vi "build memory.vi"(8 "error in (no error)":errorcluster caption="에러 입력(에러 없음)", 10 "WF List":T1[](array[typedef]), 11 "Haptic IC 입력":refnum<class "Haptic IC.lvclass">) -> (0 "error out":errorcluster caption="에러 출력", 1 "memory data by wf":cluster{"Header":u8[], "Data":u8[]}[](array[cluster]), 2 "full memory data":u8[](array[numeric]), 3 "Haptic IC 출력":refnum<class "Haptic IC.lvclass">)   [LabVIEW 2020, in "Haptic IC.lvclass"]
uses:
  Haptic IC.lvclass
  SubVIs/Waveform Editor/Controls/(Ctrl)Waveform Editor_WF List.ctl
  Waveform Obj Class/Waveform Obj/Waveform Obj.lvclass
  Waveform Obj Class/Waveform Obj/Waveform Obj.lvclass/Waveform Obj.ctl
  Waveform Obj Class/Waveform Obj/Accessors/Read sampling rate.vi
  Waveform Obj Class/Waveform Obj/Accessors/Read voltage range.vi
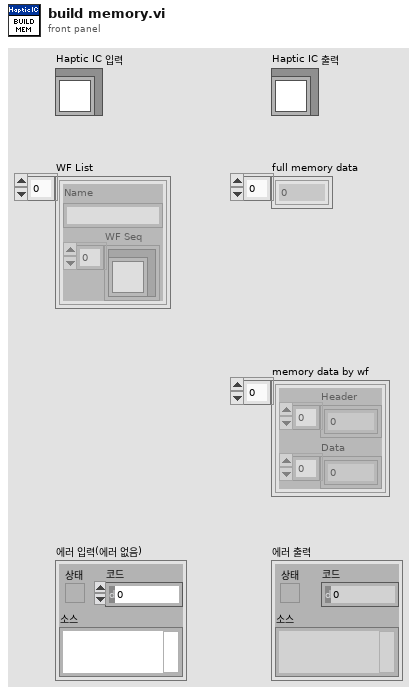
[diagram p1: front panel]
types:
  T1 = typedef "(Ctrl)Waveform Editor_WF List.ctl" = cluster{"Name":string, "WF Seq":refnum<class "Waveform Obj.lvclass">[]}
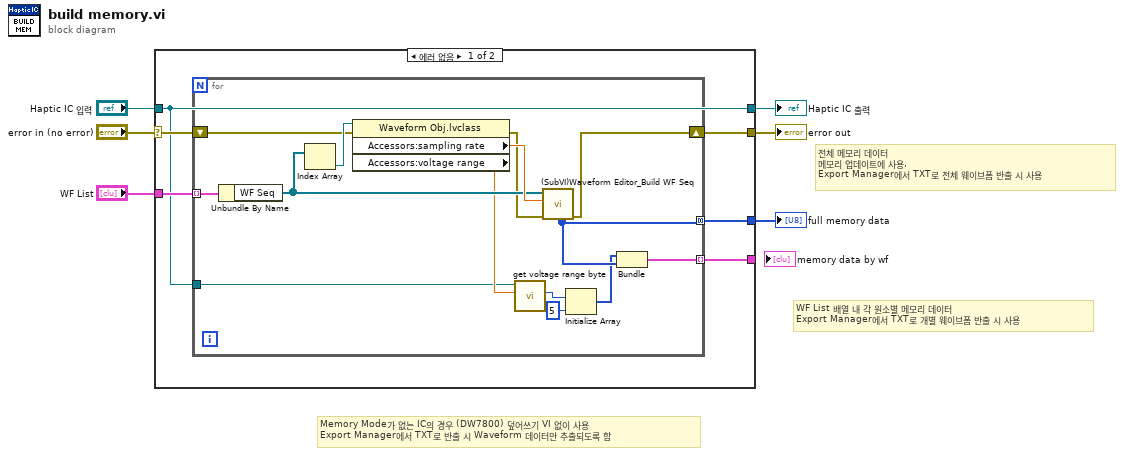
[diagram p0: block diagram]
diagram:
  # "WF List 배열 내 각 원소별 메모리 데이터\nExport Manager에서 TXT로 개별 웨이브폼 반출 시 사용"
  # "전체 메모리 데이터\n메모리 업데이트에 사용,\nExport Manager에서 TXT로 전체 웨이브폼 반출 시 사용"
  # "Memory Mode가 없는 IC의 경우 (DW7800) 덮어쓰기 VI 없이 사용\nExport Manager에서 TXT로 반출 시 Waveform 데이터만 추출되도록 함"
  n1 = case shown="에러 없음" "error in (no error)" {
    selector: "error in (no error)" -> [w11 w28]
    tunnel: [w8 w28] -> w4
    tunnel: [w7 w27] -> w5
    tunnel: "Haptic IC 입력" -> [w7 w27]
    tunnel: "WF List" -> [w12 _]
    tunnel: [w10 _] -> w1
    tunnel: [w9 _] -> _
    frame No Error {
      n2 = for {
        tunnel: w12 -> [w26] mode=indexing
        tunnel: [w18] -> w10 mode=concatenating
        tunnel: [w20] -> w9 mode=indexing
        shift-right: [w19] -> w8
        shift-left: w11 -> [w23]
        tunnel: w7 -> [w13]
        n3 = Unbundle By Name(w26) -> ("WF Seq"=w22:refnum<class "Waveform Obj.lvclass">[])
        n4 = Index Array(array=w22) -> (element=w25:refnum<class "Waveform Obj.lvclass">)  [unwired: 1 in]
        n5 = property class="Waveform Obj.lvclass"(reference=w25, error in=w23) -> (error out=w21:errorcluster, "Accessors:sampling rate"=w24:dbl, "Accessors:voltage range"=w17:dbl)  [unwired: 1 out]
        n6 = call-dynamic "get voltage range byte.vi"("voltage range"=w17, "Haptic IC 입력"=w13) -> ("byte value"=w16:u8)  [unwired: 7 in, 2 out]
        n7 = call "(SubVI)Waveform Editor_Build WF Seq.vi"("error in (no error)"=w21, "Sampling Rate"=w24, "WF Seq"=w22) -> ("error out"=w19:errorcluster, "8bit memory data"=w18:u8[])  [unwired: 3 in, 4 out]
        n8 = Initialize Array(w16, 5 ("차원 크기")) -> (w14:u8[])
        n9 = Bundle(w14, "8bit memory data"=w18) -> (w20:cluster{u8[], "8bit memory data":u8[]})  [unwired: 1 in]
      }
    }
    frame Error {
    }
  }
  "error out" <- w4
  "Haptic IC 출력" <- w5
  "full memory data" <- w1
